vi "to.net.vi"(11 "Variant":variant) -> (3 "Array":refnum<k24>[](array[refnum]))   [LabVIEW 2018, in "LVTiffWriter.lvlib"]
uses:
  LVTiffWriter.lvlib
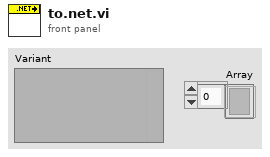
[diagram p1: front panel]
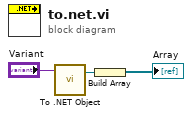
[diagram p0: block diagram]
diagram:
  n1 = call <vilib>:"To .NET Object.vi"("anything"="Variant") -> (".NET object"=w2:refnum<k24>)  [unwired: 1 in, 1 out]
  n2 = Build Array(w2) -> (→"Array":refnum<k24>[])
